vi "KernelRidge.vi"(8 "error in":errorcluster) -> (0 "error out":errorcluster, 3 "out":refnum<class "KernelRidge.lvclass">)   [LabVIEW 2020]
doc: "Kernel ridge regression.\n\n Kernel ridge regression (KRR) combines ridge regression (linear least\n squares with l2-norm regularization) with the kernel trick. It thus\n learns a linear function in the space induced by the respective kernel and\n the data. For non-linear kernels, this corresponds to a non-linear\n function in the original space.\n\n The form of the model learned by KRR is identical to support vector\n regression (SVR). However, different loss functions are used: KRR uses\n squared error loss while support vector regression uses epsilon-insensitive\n loss, both combined with l2 regularization. In contrast to SVR, fitting a\n KRR model can be done in closed-form and is typically faster for\n medium-sized datasets. On the other hand, the learned model is non-sparse\n and thus slower than SVR, which learns a sparse model for epsilon > 0, at\n prediction-time.\n\n This estimator has built-in support for multi-variate regression\n (i.e., when y is a 2d-array of shape [n_samples, n_targets]).\n\n Read more in the :ref:`User Guide <kernel_ridge>`.\n\n Parameters\n ----------\n alpha : float or array-like of shape (n_targets,), default=1.0\n Regularization strength; must be a positive float. Regularization\n improves the conditioning of the problem and reduces the variance of\n the estimates. Larger values specify stronger regularization.\n Alpha corresponds to ``1 / (2C)`` in other linear models such as\n :class:`~sklearn.linear_model.LogisticRegression` or\n :class:`~sklearn.svm.LinearSVC`. If an array is passed, penalties are\n assumed to be specific to the targets. Hence they must correspond in\n number. See :ref:`ridge_regression` for formula.\n\n kernel : string or callable, default=\"linear\"\n Kernel mapping used internally. This parameter is directly passed to\n :class:`~sklearn.metrics.pairwise.pairwise_kernel`.\n If `kernel` is a string, it must be one of the metrics\n in `pairwise.PAIRWISE_KERNEL_FUNCTIONS`.\n If `kernel` is \"precomputed\", X is assumed to be a kernel matrix.\n Alternatively, if `kernel` is a callable function, it is called on\n each pair of instances (rows) and the resulting value recorded. The\n callable should take two rows from X as input and return the\n corresponding kernel value as a single number. This means that\n callables from :mod:`sklearn.metrics.pairwise` are not allowed, as\n they operate on matrices, not single samples. Use the string\n identifying the kernel instead.\n\n gamma : float, default=None\n Gamma parameter for the RBF, laplacian, polynomial, exponential chi2\n and sigmoid kernels. Interpretation of the default value is left to\n the kernel; see the documentation for sklearn.metrics.pairwise.\n Ignored by other kernels.\n\n degree : float, default=3\n Degree of the polynomial kernel. Ignored by other kernels.\n\n coef0 : float, default=1\n Zero coefficient for polynomial and sigmoid kernels.\n Ignored by other kernels.\n\n kernel_params : mapping of string to any, default=None\n Additional parameters (keyword arguments) for kernel function passed\n as callable object.\n\n Attributes\n ----------\n dual_coef_ : ndarray of shape (n_samples,) or (n_samples, n_targets)\n Representation of weight vector(s) in kernel space\n\n X_fit_ : {ndarray, sparse matrix} of shape (n_samples, n_features)\n Training data, which is also required for prediction. If\n kernel == \"precomputed\" this is instead the precomputed\n training matrix, of shape (n_samples, n_samples).\n\n References\n ----------\n * Kevin P. Murphy\n \"Machine Learning: A Probabilistic Perspective\", The MIT Press\n chapter 14.4.3, pp. 492-493\n\n See Also\n --------\n sklearn.linear_model.Ridge : Linear ridge regression.\n sklearn.svm.SVR : Support Vector Regression implemented using libsvm.\n\n \nAvailable methods:\nGet Attributes\nGet Params\nSet Params"
uses:
  KernelRidge/KernelRidge.lvclass
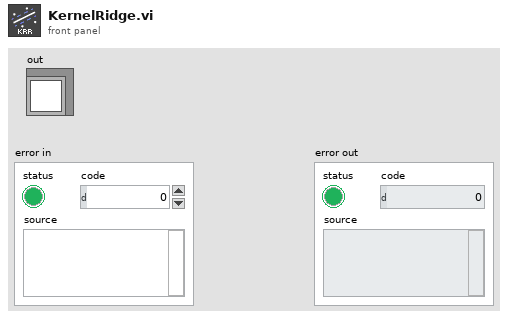
[diagram p1: front panel]
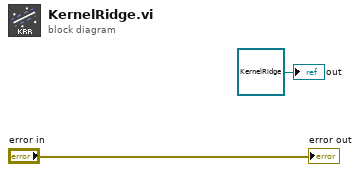
[diagram p0: block diagram]
diagram:
  "out" <- refnum<class "KernelRidge.lvclass"> refnum ("model")
  "error out" <- "error in"
